vi "sub_main_DS1202.vi"(8 "error in":errorcluster) -> (0 "error out":errorcluster)   [LabVIEW 2021]
uses:
  ctrl/create-rw-close.ctl
  ctrl/hw-lists.ctl
  ctrl/DS1202_cmd.ctl
  ctrl/ini-stop-read.ctl
  ctrl/5110_q.ctl
panel:
  out "Numeric 2":i32
  out "Numeric":i32
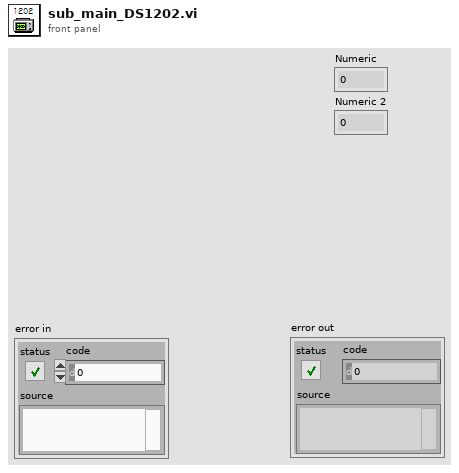
[diagram p1: front panel]
types:
  T1 = typedef "hw-lists.ctl" = enum16{"PXIe-5110", "PXIe-5413", "PXIe-2530", "DS1202"}
  T2 = typedef "create-rw-close.ctl" = enum16{"create", "read", "write", "close"}
  T3 = typedef "DS1202_cmd.ctl" = enum16{"init", "auto", "read", "close"}
  T4 = typedef "5110_q.ctl" = enum16{"create", "read", "write", "close"}
  T5 = typedef "ini-stop-read.ctl" = enum16{"init", "stop", "read"}
  T6 = typedef "run-check-stop.ctl" = enum16{"run", "check", "stop"}
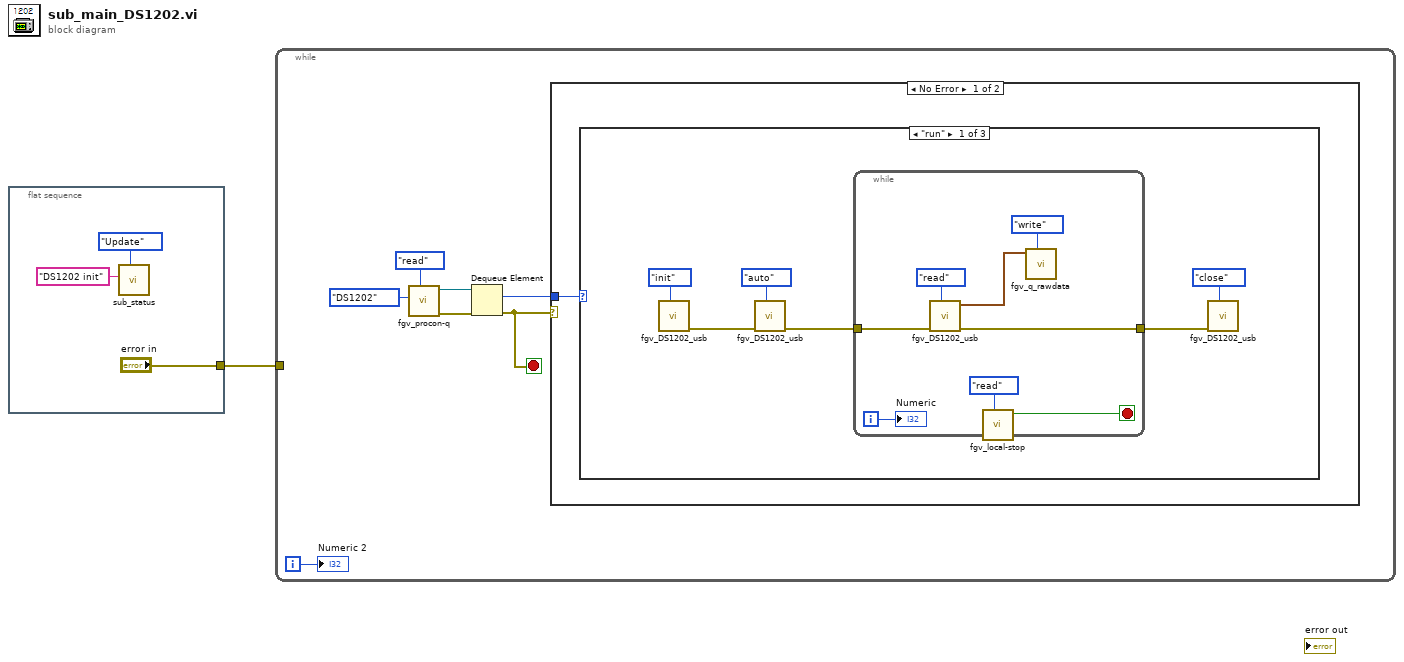
[diagram p0: block diagram]
diagram:
  n1 = flat-sequence {
    tunnel: ["error in"] -> w1
    frame #0 {
      n2 = call "sub_status.vi"("Mode"=enum16{"Initial", "Update", "Clear"}."Update", "title"="DS1202 init") -> ()  [unwired: 9 in, 1 out]
    }
  }
  n3 = while {
    tunnel: w1 -> [_]
    i -> [w5]
    stop <- w6 stop-if-true
    n4 = call "fgv_procon-q.vi"("cmd 2"=create-rw-close."read", "hw lists"=hw-lists."DS1202") -> ("error out"=w10:errorcluster, "ref"=w11:refnum<queue>)  [unwired: 7 in, 1 out]
    n5 = Dequeue Element(queue=w11, error in (no error)=w10) -> (element=w7:T6, error out=w6:errorcluster)  [unwired: 1 in, 2 out]
    n6 = case shown="No Error" w6 {
      tunnel: w7 -> [w12 _]
      frame No Error {
        n7 = case shown="\"run\"" w12 {
          frame "run" {
            n8 = call "fgv_DS1202_usb.vi"("cmd"=DS1202_cmd."init") -> ("error out"=w16:errorcluster)  [unwired: 9 in, 1 out]
            n9 = call "fgv_DS1202_usb.vi"("cmd"=DS1202_cmd."auto", "error in"=w16) -> ("error out"=w14:errorcluster)  [unwired: 8 in, 1 out]
            n10 = while {
              tunnel: w14 -> [w25]
              tunnel: [w24] -> w13
              i -> [w19]
              stop <- w22 stop-if-true
              n11 = call "fgv_DS1202_usb.vi"("cmd"=DS1202_cmd."read", "error in"=w25) -> ("error out"=w24:errorcluster, "wfm"=w20:waveform(dbl))  [unwired: 8 in]
              n12 = call "fgv_local-stop.vi"("cmd"=ini-stop-read."read") -> ("stop"=w22:bool)  [unwired: 10 in]
              n13 = call "fgv_q_rawdata.vi"("cmd"=5110_q."write", "wfm"=w20) -> ()  [unwired: 8 in, 2 out]
              "Numeric" <- w19
            }
            n14 = call "fgv_DS1202_usb.vi"("cmd"=DS1202_cmd."close", "error in"=w13) -> ()  [unwired: 8 in, 2 out]
          }
          frame "check" {
          }
          frame "stop", Default {
          }
        }
      }
      frame Error {
      }
    }
    "Numeric 2" <- w5
  }
